vi "emi_Init application.vi"(5 "System ID(0)":u8, 11 "error in (no error)":errorcluster, 12 "Version Info in":T1={"Name"="Default Name", "Major"=0, "Minor"=0, "Fix"=0, "Build"=0, "Type"=enum."Alfa", "Dev"=FALSE, "Version Name"="", "Date"=timestamp(0 s since 1904-01-01)} {"Date" format="%<%y%m%d>T"}) -> (15 "error out":errorcluster)   [LabVIEW 2011]
doc: "Initialises the sys01 parts of an application as needed.\n\nRegisters version, \nRegisters system ID\nrecords program starte dmessage(Note id 0)"
uses:
  Basic/0 - General/App/Version/Private/emi_Version Info.ctl
  Host Code/Application Structure/E&S Note ID.ctl
  Host Code/emi cndiates/E&S/reate/S&E Event source.ctl
  emi_Read System ID.vi
  Private/_emi_GFV System ID.vi
  <vilib>/Utility/error.llb/Clear Errors.vi
  S&E reporting/Private/_emi_S&E Q Generator.vi
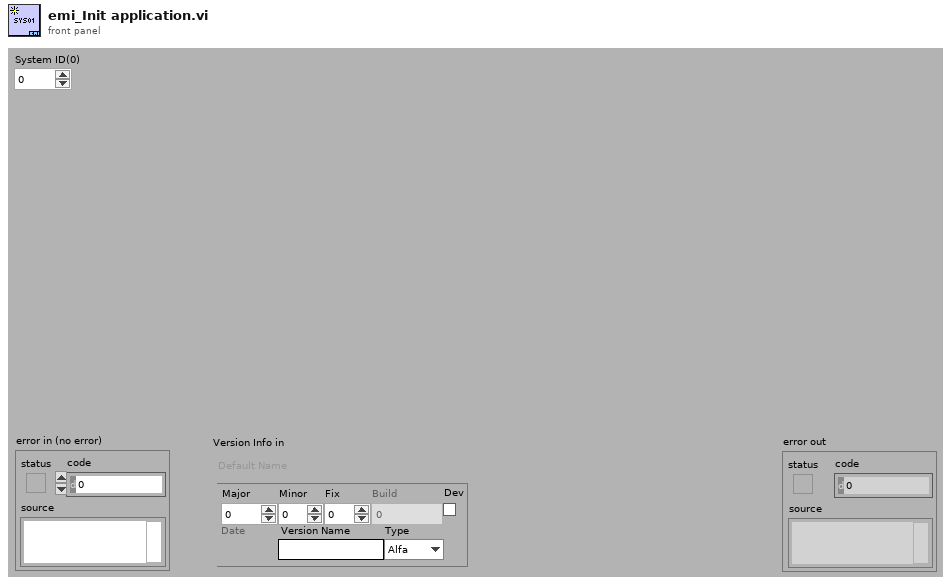
[diagram p1: front panel]
types:
  T1 = typedef "emi_Version Info.ctl" = cluster{"Name":string, "Major":i16, "Minor":i16, "Fix":i16, "Build":i32, "Type":enum16{"Alfa", "Beta", "Stable"}, "Dev":bool, "Version Name":string, "Date":timestamp}
  T2 = typedef "S&E Event source.ctl" = enum16{"User", "Instrument", "Application", "Windows"}
  T3 = typedef "E&S Note ID.ctl" = enum16{"Program Started", "Program terminated", "User Changed", "General information"}
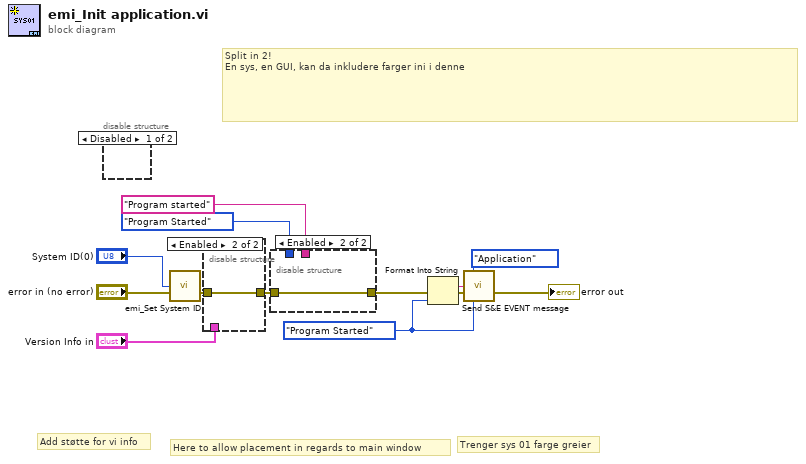
[diagram p0: block diagram]
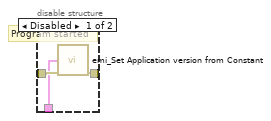
[diagram p2: hidden frame]
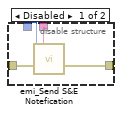
[diagram p3: hidden frame]
diagram:
  w4 = enum16{"Program Started", "Program Ending"}."Program Started" ("App Events")
  # "Split in 2! \nEn sys, en GUI, kan da inkludere farger ini i denne"
  # "Trenger sys 01 farge greier"
  # "Here to allow placement in regards to main window"
  # "Add støtte for vi info"
  n1 = disable-structure shown="Disabled" {
    frame Disabled {
    }
    frame Enabled {
    }
  }
  n2 = call "emi_Set System ID.vi"("System ID(0)"="System ID(0)", "error in (no error)"="error in (no error)") -> ("error out"=w13:errorcluster)  [unwired: 13 in]
  n3 = disable-structure shown="Enabled" {
    disable-tunnel: w13 -> [w16 w17]
    disable-tunnel: [w15 w17] -> w12
    disable-tunnel: "Version Info in" -> [w14 _]
    frame Disabled {
      # "Program started"
      n4 = call "emi_Set Application version from Constant.vi"("Version Info in"=w14, "error in (no error)"=w16) -> ("error out"=w15:errorcluster)  [unwired: 12 in, 1 out]
    }
    frame Enabled {
    }
  }
  n5 = disable-structure shown="Enabled" {
    disable-tunnel: w12 -> [w21 w22]
    disable-tunnel: [w20 w22] -> w3
    disable-tunnel: E&S_Note_ID."Program Started" ("E&S note ID") -> [w19 _]
    disable-tunnel: "Program started" ("Note(\"\")") -> [w18 _]
    frame Disabled {
      n6 = call "emi_Send S&E Notefication.vi"("Note(\"\")"=w18, 7:w19, "error in (no error)"=w21) -> ("error out"=w20:errorcluster)  [unwired: 11 in, 1 out]
    }
    frame Enabled {
    }
  }
  n7 = Format Into String(error in=w3, w4) -> (resulting string=w1:string, error out=w2:errorcluster)  [unwired: 2 in]
  n8 = call "Send S&E EVENT message.vi"("Event Source(user)"=S&E_Event_source."Application", "Event Description"=w1, "error in (no error)"=w2, "Loc Sub ID/Event ID(No ID)"=w4) -> ("error out"=→"error out":errorcluster)  [unwired: 10 in, 1 out]
